vi "drawcarroad.vi"   [LabVIEW 2013]
uses:
  <vilib>/NXT/Dual Mode Library/Display/drawPicture.vi
  <vilib>/NXT/Dual Mode Library/Waits/Wait_Num.vi
types:
  T1 = typedef "LVHSConnector.ctl" = refnum<class "BrickReference.lvclass">
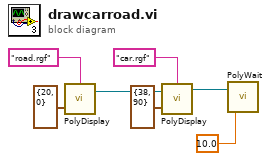
[diagram p0: block diagram]
diagram:
  n1 = call-poly <vilib>:"PolyDisplay.vi"("Origin"=cluster{"X":i16, "Y":i16} {"X"=20, "Y"=0}, "Filename (*.ric/*.rgf)"="road.rgf") -> ("NXT/EV3"=w7:T1)  [unwired: 2 in]
  n2 = call-poly <vilib>:"PolyDisplay.vi"("Origin"=cluster{"X":i16, "Y":i16} {"X"=38, "Y"=90}, "NXT/EV3"=w7, "Filename (*.ric/*.rgf)"="car.rgf") -> ("NXT/EV3"=w4:T1)  [unwired: 1 in]
  n3 = call-poly <vilib>:"PolyWait.vi"("Time (1 sec)"=sgl 10.0, "NXT/EV3"=w4) -> ()  [unwired: 2 in, 1 out]
